vi "JL_Obtain Time LED Config.vi"(0 "Time Option":u8 format="%x") -> (4 "Fail":bool, 6 "Pass":bool, 8 "Time Setting":T1)   [LabVIEW 2016]
uses:
  type defs/Time Enum.ctl
panel:
  # "All integers are hex"
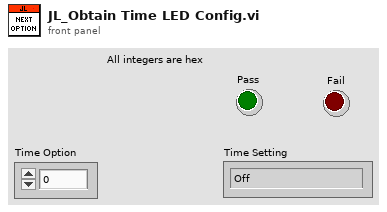
[diagram p1: front panel]
types:
  T1 = typedef "Time Enum.ctl" = enum16{"Off", "Default Time 1", "Default Time 2", "Default Time 3", "Default Time 4", "Default Time 5", "*Incorrect*"}
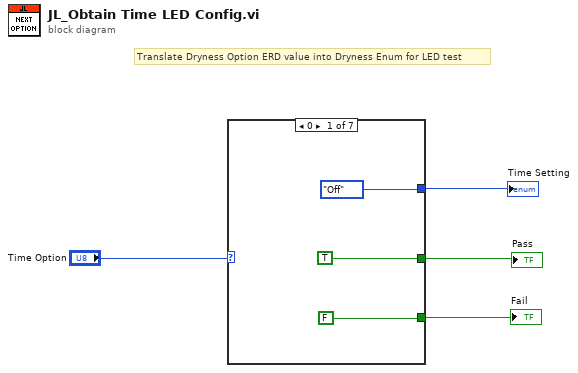
[diagram p0: block diagram]
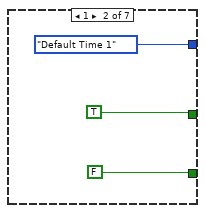
[diagram p2: hidden frame]
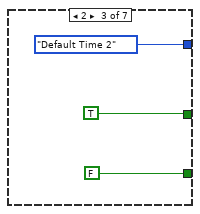
[diagram p3: hidden frame]
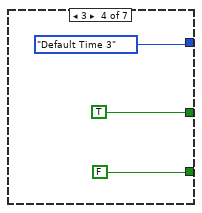
[diagram p4: hidden frame]
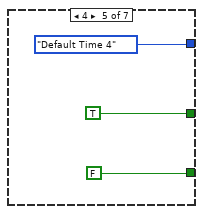
[diagram p5: hidden frame]
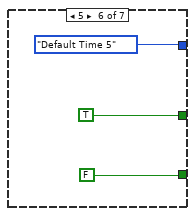
[diagram p6: hidden frame]
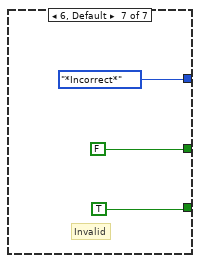
[diagram p7: hidden frame]
diagram:
  # "Translate Dryness Option ERD value into Dryness Enum for LED test"
  n1 = case shown="0" "Time Option" {
    tunnel: [Time_Enum."Off" ("Time Setting 2") Time_Enum."Default Time 1" ("Time Setting 2") Time_Enum."Default Time 2" ("Time Setting 2") Time_Enum."Default Time 3" ("Time Setting 2") Time_Enum."Default Time 4" ("Time Setting 2") Time_Enum."Default Time 5" ("Time Setting 2") Time_Enum."*Incorrect*" ("Time Setting 2")] -> w1
    tunnel: [TRUE ("Pass 2") TRUE ("Pass 2") TRUE ("Pass 2") TRUE ("Pass 2") TRUE ("Pass 2") TRUE ("Pass 2") FALSE ("Pass 2")] -> w3
    tunnel: [FALSE ("Pass 2") FALSE ("Pass 2") FALSE ("Pass 2") FALSE ("Pass 2") FALSE ("Pass 2") FALSE ("Pass 2") TRUE ("Pass 2")] -> w2
    frame 0 {
    }
    frame 1 {
    }
    frame 2 {
    }
    frame 3 {
    }
    frame 4 {
    }
    frame 5 {
    }
    frame 6, Default {
      # "Invalid"
    }
  }
  "Pass" <- w3
  "Fail" <- w2
  "Time Setting" <- w1
